vi "Split Command Prefix.vi"(0 "command string in":string, 11 "error in":errorcluster) -> (4 "command prefix":string, 6 "command out":string, 15 "error out":errorcluster)   [LabVIEW 2019, in "mmW_commands.lvlib"]
doc: "input format : \"prefix:command\"\n\nReturns error if split was unsuccessful."
uses:
  mmW_commands.lvlib
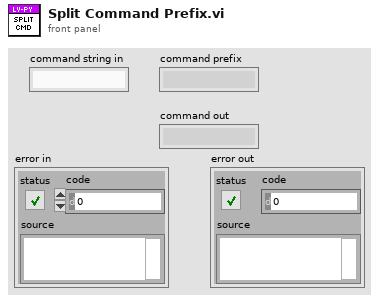
[diagram p1: front panel]
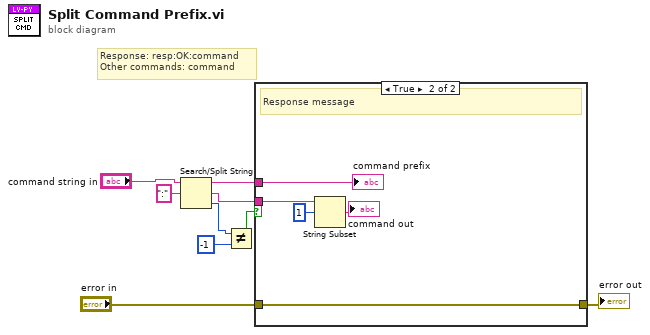
[diagram p0: block diagram]
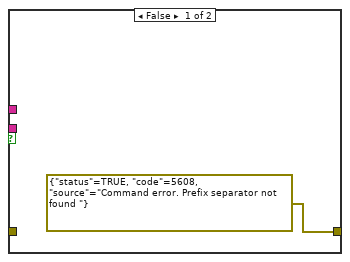
[diagram p2: hidden frame]
diagram:
  # "Response: resp:OK:command\nOther commands: command"
  n1 = Search/Split String(string="command string in", search string/char (-)=":") -> (substring before match=w9:string, match + rest of string=w7:string, offset of match=w4:i32)  [unwired: 1 in]
  n2 = Not Equal?(x=w4, y=-1) -> (x != y?=w3:bool)
  n3 = case shown="True" w3 {
    tunnel: w9 -> [_ w15]
    tunnel: w7 -> [_ w12]
    tunnel: "error in" -> [_ w11]
    tunnel: [errorcluster {"status"=TRUE, "code"=5608, "source"="Command error. Prefix separator not found "} ("error in") w11] -> w1
    frame False {
    }
    frame True {
      # "Response message"
      n4 = String Subset(string=w12, offset (0)=1) -> (substring=→"command out":string)  [unwired: 1 in]
      "command prefix" <- w15
    }
  }
  "error out" <- w1
